vi "aal_cascaded moving average (real input).vi"(1 "Reset":bool, 2 "Stages":i32=1, 3 "N":i32=2, 4 "x":dbl[](array[numeric])) -> (0 "y":dbl[](array[numeric]))   [LabVIEW 2017, in "NI_AALPro.lvlib"]
uses:
  NI_AALPro.lvlib
  lvanlys.dll
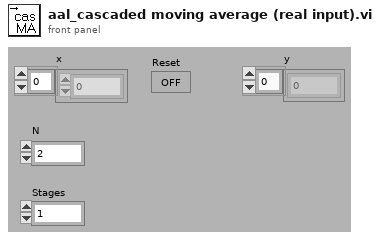
[diagram p1: front panel]
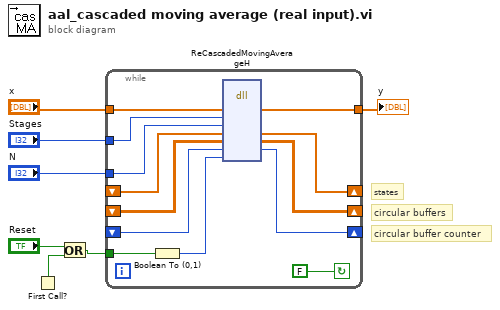
[diagram p0: block diagram]
diagram:
  # "circular buffer counter"
  # "circular buffers"
  # "states"
  n1 = First Call?() -> (First Call?: T/F=w3:bool)
  n2 = Or(x="Reset", y=w3) -> (x .or. y?=w4:bool)
  n3 = while {
    tunnel: w4 -> [w8]
    tunnel: "x" -> [w9]
    tunnel: [w10] -> w1
    tunnel: "Stages" -> [w13]
    tunnel: "N" -> [w14]
    shift-left: _ -> [w18]
    shift-right: [w17] -> _
    shift-left: _ -> [w15]
    shift-right: [w16] -> _
    shift-left: _ -> [w20]
    shift-right: [w19] -> _
    stop <- FALSE continue-if-true
    n4 = Boolean To (0,1)(Boolean=w8) -> (0, 1=w12:i16)
    n5 = dll-call lib="C:/Program Files/National Instruments/LabVIEW 2017/resource/lvanlys.*" fn="ReCascadedMovingAverageH"("x"=w9, "stages"=w13, "N"=w14, "states"=w20, "ibuf"=w18, "ibuf_cnt"=w15, "Reset"=w12) -> ("x"=w10:dbl[], "states"=w19:dbl[], "ibuf"=w17:dbl[][], "ibuf_cnt"=w16:i32)  [unwired: 7 in, 2 out]
  }
  "y" <- w1
